vi "Packet Decode.vi"(8 "error in (no error)":errorcluster, 10 "Data":u8[](array[numeric]), 11 "Score in":refnum<class "Score.lvclass">) -> (0 "error out":errorcluster, 3 "Score out":refnum<class "Score.lvclass">)   [LabVIEW 2019, in "Score.lvclass"]
uses:
  Score.lvclass
  PlayerUpdate/PlayerUpdate.lvclass
  TCP Packet/Packet.lvclass
  C:/projects/labview_multiplayer_snake/Main Codeline/Software/Code/Shared/PlayerUpdate/PlayerUpdate.lvclass
  C:/projects/labview_multiplayer_snake/Main Codeline/Software/Code/Shared/TCP/JSONPayload/JSONPayload.lvclass
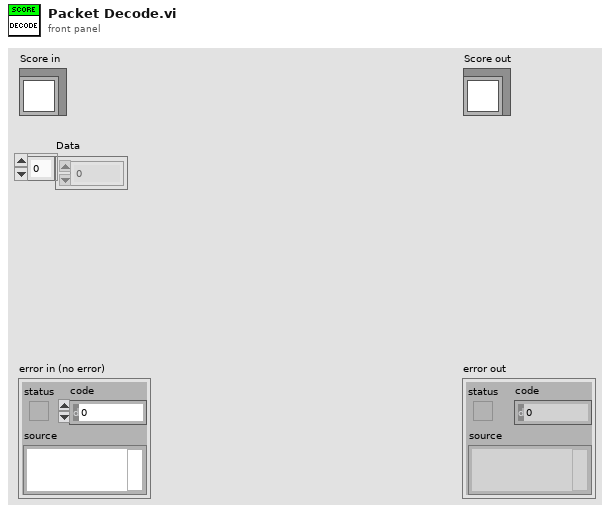
[diagram p1: front panel]
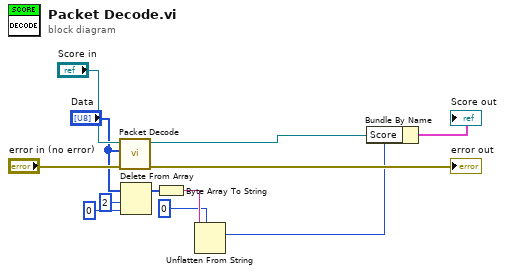
[diagram p0: block diagram]
diagram:
  n1 = call-parent "Packet Decode.vi"("error in (no error)"="error in (no error)", "Data"="Data", "Packet in"="Score in") -> ("error out"=→"error out":errorcluster, "Packet out"=w11:refnum<class "Packet.lvclass">)  [unwired: 7 in]
  n2 = Delete From Array(array="Data", length=2, index=0) -> (array with subset deleted=w4:u8[])  [unwired: 1 out]
  n3 = Byte Array To String(unsigned byte array=w4) -> (string=w3:string)
  n4 = Unflatten From String(type=u32 0, binary string=w3) -> (value=w1:u32)  [unwired: 3 in, 2 out]
  n5 = Bundle By Name(cluster=w11, "Score"=w1) -> (→"Score out":cluster{})
